vi "re_LuaVIEW Incite.vi"(0 "task":string, 1 "timeout [ms] (use default)":u32, 5 "LuaVIEW reference in":T1, 11 "error in (no error)":errorcluster) -> (4 "reply":string, 6 "LuaVIEW reference out":T1, 15 "error out":errorcluster)   [LabVIEW 2012]
doc: "Incite a task to send a reply. This is done by sending the task to be incited a message containing the task identifier of the current task. The incited task can then perform whatever service it is designed to provide and use that identifier to send a reply message when it is done. This VI returns on receiving the reply unless an error occurs.\n\nAn error occurs when the provided LuaVIEW reference is not associated with a task (this VI is not called inside a task) or when the task being incited does not exist, is in error mode, or fails to reply before the timeout expires. BEWARE: the task doing the incitation should not be receiving other types of messages at the same time lest these get confused with the incitation reply.\n\nIncitation provides an easy means of synchronously using a service provided by an asynchronous task. More complex message/reply mechanisms can be coded in similar fashion: this VI merely constitutes a convenience implementation of the instigating side of the simplest conceivable message/reply mechanism. Module export functions also allow a synchronous service to be offered and involve less overhead on account of not requiring a context switch. The advantage of a message/reply mechanism is that the service can be implemented as a task script that can also add asynchronous actions such as periodic updates into the mix."
uses:
  typedefs/t_LuaVIEW Reference.ctl
  typedefs/t_LuaVIEW Task State Methods.ctl
  typedefs/t_LuaVIEW Task List Methods.ctl
  glb_LuaVIEW Configuration Globals.vi
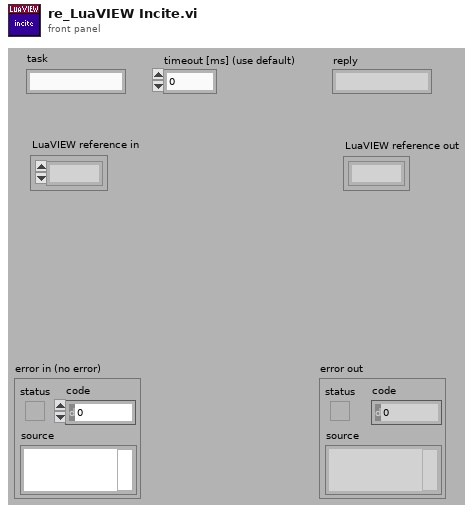
[diagram p1: front panel]
types:
  T1 = typedef "t_LuaVIEW Reference.ctl" = refnum<k1>
  T2 = typedef "t_LuaVIEW Task State Methods.ctl" = enum16{"cleanup", "set initial", "set mode", "set active mode", "set error", "get task info", "get script info", "set signal", "clear signal", "test handled", "test delegated", "test signal", "handle signal", "delegate signal", "allow signal", "disallow signal", "disallow all", "signals?", "delegated signals?", "protection++", "protection--", "protection=0", "message", "next message", "pop message", "message available?", "force stop", "set swap preps", "apply swap preps"}
  T3 = typedef "t_LuaVIEW Task List Methods.ctl" = enum16{"clear list", "add", "test", "remove", "get ref", "get task info", "get list", "get script info", "ongoing?", "resume", "pause", "stop", "confirm", "message"}
  T4 = typedef "t_LuaVIEW Task State Pane.ctl" = refnum<vi>
  T5 = typedef "LuaVIEW Task Info.ctl" = cluster{"main script":string, "identifier":string, "class":string, "description":string, "mode":T6, "handler":string, "LuaVIEW reference":T1, "scripts":i32, "hide":bool, "active":bool, "error msg":string, "defer":bool, "launch":enum16{"asynchronous", "manual", "synchronous"}, "main path valid":bool, "start time":dbl, "swap time":dbl, "task VI":refnum<vi>, "prefsys":enum32{"invalid execution system", "user interface", "standard", "instrument i/o", "data acquisition", "other 1", "other 2", "same as caller"}, "priority":enum32{"invalid priority", "background priority", "normal priority", "above normal priority", "high priority", "time critical priority", "subroutine"}, "signal flags":u32, "allow mask":u32, "handle mask":u32, "disallow manual":bool}
  T6 = typedef "t_LuaVIEW Task Modes.ctl" = enum16{"initializing", "running", "executing", "paused", "error", "swapping"}
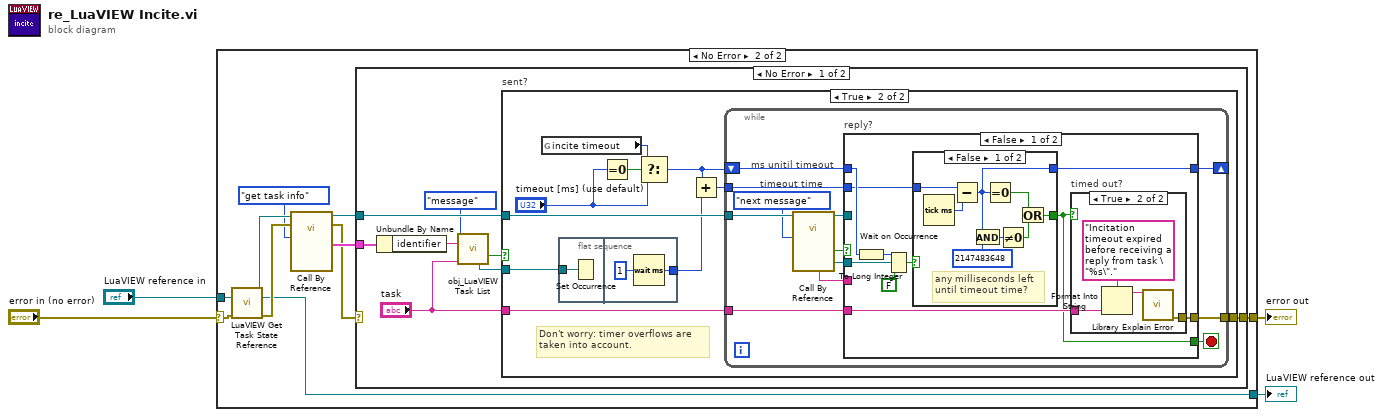
[diagram p0: block diagram]
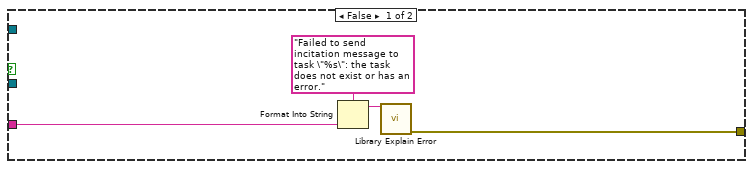
[diagram p3: hidden frame]
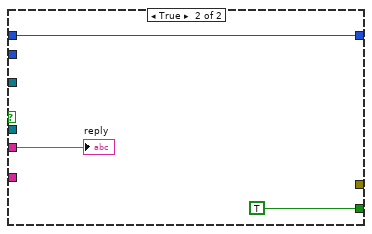
[diagram p6: hidden frame]
diagram:
  n1 = case shown="No Error" "error in (no error)" {
    selector: "error in (no error)" -> [w6 w16]
    tunnel: [w5 w7] -> w1
    tunnel: "LuaVIEW reference in" -> [w5 w15]
    tunnel: [w6 w9] -> w3
    frame Error {
    }
    frame No Error {
      n2 = call "LuaVIEW Get Task State Reference.vi"("LuaVIEW reference in"=w15, "error in (no error)"=w16) -> ("task state reference"=w14:T4, "LuaVIEW reference out"=w7:T1, "error out"=w13:errorcluster)  [unwired: 11 in]
      n3 = call-by-ref "?"(reference=w14, error in=w13, "method"=t_LuaVIEW_Task_State_Methods."get task info") -> (reference out=w8:T4, error out=w10:errorcluster, "task info {get task info}"=w11:T5)  [unwired: 10 in, 4 out]
      n4 = case shown="No Error" w10 {
        selector: w10 -> [_ w80]
        tunnel: w11 -> [w24 _]
        tunnel: [w21 w80] -> w9
        tunnel: w8 -> [w22 _]
        frame No Error {
          n5 = Unbundle By Name(w24) -> ("identifier"=w23:string)
          n6 = call "obj_LuaVIEW Task List.vi"("method"=t_LuaVIEW_Task_List_Methods."message", "message"=w23, "task identifier"="task") -> ("set/ongoing"=w19:bool, "wakeup occurrence"=w17:refnum<k4>)  [unwired: 7 in, 4 out]
          n7 = case "sent?" shown="True" w19 {
            tunnel: w22 -> [_ w38]
            tunnel: [w25 w36] -> w21
            tunnel: "task" -> [w26 w37]
            tunnel: w17 -> [_ w29]
            frame False {
              n8 = Format Into String(format string="Failed to send incitation message to task \"%s\": the task does not exist or has an error.", w26) -> (resulting string=w28:string)  [unwired: 2 in, 1 out]
              n9 = call "Library Explain Error.vi"("explanation prefix (none)"=w28) -> ("explained error"=w25:errorcluster)  [unwired: 14 in]
            }
            frame True {
              # "Don't worry: timer overflows are\ntaken into account."
              n10 = global read "glb_LuaVIEW Configuration Globals.vi" "incite timeout"() -> (w34:u32)
              n11 = flat-sequence {
                tunnel: w29 -> [w39]
                tunnel: [w40] -> w30
                frame #0 {
                  n12 = Set Occurrence(w39) -> ()
                }
                frame #1 {
                  n13 = Wait (ms)(milliseconds to wait=u32 1) -> (millisecond timer value=w40:u32)
                }
              }
              n14 = Equal To 0?(x="timeout [ms] (use default)") -> (x = 0?=w35:bool)
              n15 = Select(t=w34, s=w35, f="timeout [ms] (use default)") -> (s? t:f=w31:u32)
              n16 = Add(x=w31, y=w30) -> (x+y=w32:u32)
              n17 = while {
                tunnel: w38 -> [w53]
                tunnel: w37 -> [w47]
                tunnel: [w46] -> w36
                shift-right: [w42] -> _
                shift-left: w31 -> [w44]
                tunnel: w32 -> [w43]
                stop <- w48 stop-if-true
                # "ms unitil timeout"
                # "timeout time"
                n18 = call-by-ref "?"(reference=w53, "method"=t_LuaVIEW_Task_State_Methods."next message") -> (reference out=w49:T4, "set/available/pending"=w51:bool, "string out"=w45:string, "wakeup occurrence"=w50:refnum<k4>)  [unwired: 11 in, 3 out]
                n19 = case "reply?" shown="False" w51 {
                  tunnel: w50 -> [w59 _]
                  tunnel: w49 -> [_ _]
                  tunnel: [w54 TRUE] -> w48
                  tunnel: w47 -> [w55 _]
                  tunnel: [w56 _] -> w46
                  tunnel: w45 -> [_ w78]
                  tunnel: w44 -> [w61 w77]
                  tunnel: w43 -> [w58 _]
                  tunnel: [w57 w77] -> w42
                  frame False {
                    n20 = To Long Integer(number=w61) -> (32bit integer=w60:i32)
                    n21 = Wait on Occurrence(1:FALSE ("ignore previous (T)"), 2:w59, 3:w60) -> (0:w62:bool)
                    n22 = case shown="False" w62 {
                      selector: w62 -> [_ w76]
                      tunnel: w58 -> [w75 _]
                      tunnel: [w72 _] -> w57
                      tunnel: [w68 w76] -> w54
                      frame False {
                        # "any milliseconds left\nuntil timeout time?"
                        n23 = Tick Count (ms)() -> (millisecond timer value=w74:u32)
                        n24 = Subtract(x=w75, y=w74) -> (x-y=w72:u32)
                        n25 = And(x=w72, y=u32 2147483648 ("x-y")) -> (x .and. y?=w71:u32)
                        n26 = Equal To 0?(x=w72) -> (x = 0?=w69:bool)
                        n27 = Not Equal To 0?(x=w71) -> (x != 0?=w70:bool)
                        n28 = Or(x=w69, y=w70) -> (x .or. y?=w68:bool)
                      }
                      frame True {
                      }
                    }
                    n29 = case "timed out?" shown="True" w54 {
                      tunnel: [_ w65] -> w56
                      tunnel: w55 -> [_ w64]
                      frame False {
                      }
                      frame True {
                        n30 = Format Into String(format string="Incitation timeout expired before receiving a reply from task \"%s\".", w64) -> (resulting string=w67:string)  [unwired: 2 in, 1 out]
                        n31 = call "Library Explain Error.vi"("explanation prefix (none)"=w67) -> ("explained error"=w65:errorcluster)  [unwired: 14 in]
                      }
                    }
                  }
                  frame True {
                    "reply" <- w78
                  }
                }
              }
            }
          }
        }
        frame Error {
        }
      }
    }
  }
  "error out" <- w3
  "LuaVIEW reference out" <- w1
